vi "MsgBox.vi"() -> ()   [LabVIEW 2020]
panel:
  out "MB":string
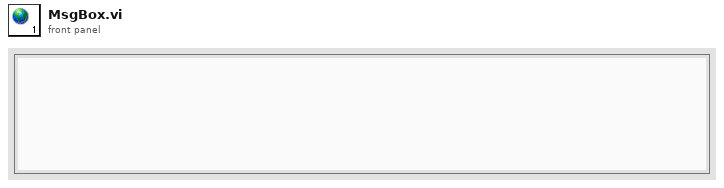
[diagram p1: front panel]
diagram:
